vi "Build And Cache Output Folder Absolute Path.vi"(0 "Sequence File Path":path, 11 "error in (no error)":errorcluster) -> (15 "error out":errorcluster)   [LabVIEW 2023, in "RFFixtureCharact.Public.lvlib"]
uses:
  RFFixtureCharact.Public.lvlib
  Common/Data Cache/Settings Dictionary/Setting Keys.vi
  Common/RFCalAndFixtureCharact.Common.lvlib
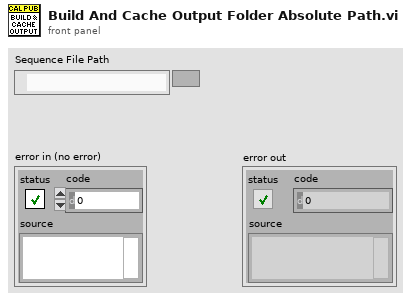
[diagram p1: front panel]
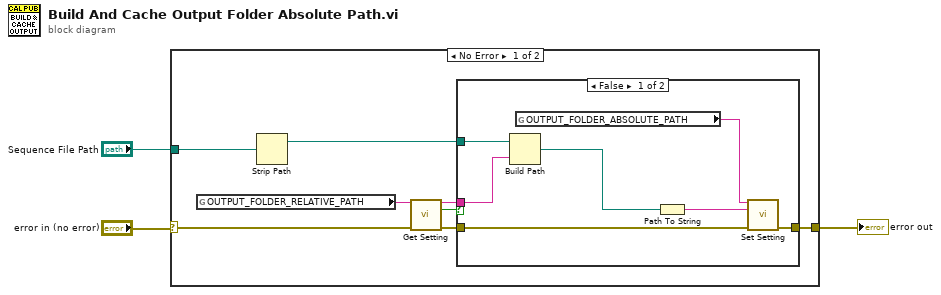
[diagram p0: block diagram]
diagram:
  n1 = case shown="No Error" "error in (no error)" {
    selector: "error in (no error)" -> [w10 w20]
    tunnel: [w11 w20] -> w2
    tunnel: "Sequence File Path" -> [w5 _]
    frame No Error {
      n2 = global read "Setting Keys.vi" "OUTPUT_FOLDER_RELATIVE_PATH"() -> (w6:string)
      n3 = Strip Path(path=w5) -> (stripped path=w4:path)  [unwired: 1 out]
      n4 = call "Get Setting.vi"("Setting name"=w6, "error in (no error)"=w10) -> ("Setting value out"=w7:string, "Setting empty or not found?"=w8:bool, "error out"=w9:errorcluster)  [unwired: 11 in]
      n5 = case shown="False" w8 {
        tunnel: w4 -> [w18 _]
        tunnel: [w15 w19] -> w11
        tunnel: w9 -> [w17 w19]
        tunnel: w7 -> [w16 _]
        frame False {
          n6 = Build Path(base path=w18, name or relative path=w16) -> (appended path=w13:path)
          n7 = global read "Setting Keys.vi" "OUTPUT_FOLDER_ABSOLUTE_PATH"() -> (w14:string)
          n8 = Path To String(path=w13) -> (string=w12:string)
          n9 = call "Set Setting.vi"("Setting name"=w14, "Setting value"=w12, "error in (no error)"=w17) -> ("error out"=w15:errorcluster)  [unwired: 10 in, 2 out]
        }
        frame True {
        }
      }
    }
    frame Error {
    }
  }
  "error out" <- w2
